vi "期末9-2.vi"() -> ()   [LabVIEW 2014]
uses:
  <vilib>/vision/NI_Vision_Development_Module.lvlib
panel:
  out "Image Out 2":T1(plugin-control)
  out "ROI":T2
  in  "紀錄中點座標和":bool
  out "填入飽和磁場分量尖點座標和 2":dbl
  out "填入飽和磁場分量尖點座標和平均 2":dbl
  in  "3. Number of Erosion":i32=10
  out "Image Out":T1(plugin-control)
  in  "紀錄電流":dbl[](array[numeric])
  in  "Tab Control 2":enum32{"座標", "座標和", "作圖"}(tab)
  out "瞬間尖點座標":dbl[][](array[numeric])
  out "尖點座標和":dbl[](array[numeric])
  out "相減結果":dbl[](array[numeric])
  out "分量-電流":cluster{"紀錄電流":dbl[], dbl[]}(graph)
  in  "紀錄":bool
  in  "結束實驗":bool
  in  "1. 範圍選擇":T3={"色相（H）"={0, 255}, "飽和度（S）"={0, 255}, "亮度（L）"={0, 255}} {"亮度（L）" scale=0.0..255.0; "飽和度（S）" scale=0.0..255.0; "色相（H）" scale=0.0..255.0}
  out "Number of Particles":i32
  out "output cluster":cluster{"X":dbl, "Y":dbl}
  in  "Tab Control":T4(tab)
  out "1. 顏色選取":T1(plugin-control)
  out "2. 填補空隙":T1(plugin-control)
  out "3. 移除雜點":T1(plugin-control)
  out "4. 形狀修正":T1(plugin-control)
  out "5. 選取結果":T1(plugin-control)
  out "Particle Measurements":dbl[][](array[numeric])
  out "Error Out":errorcluster
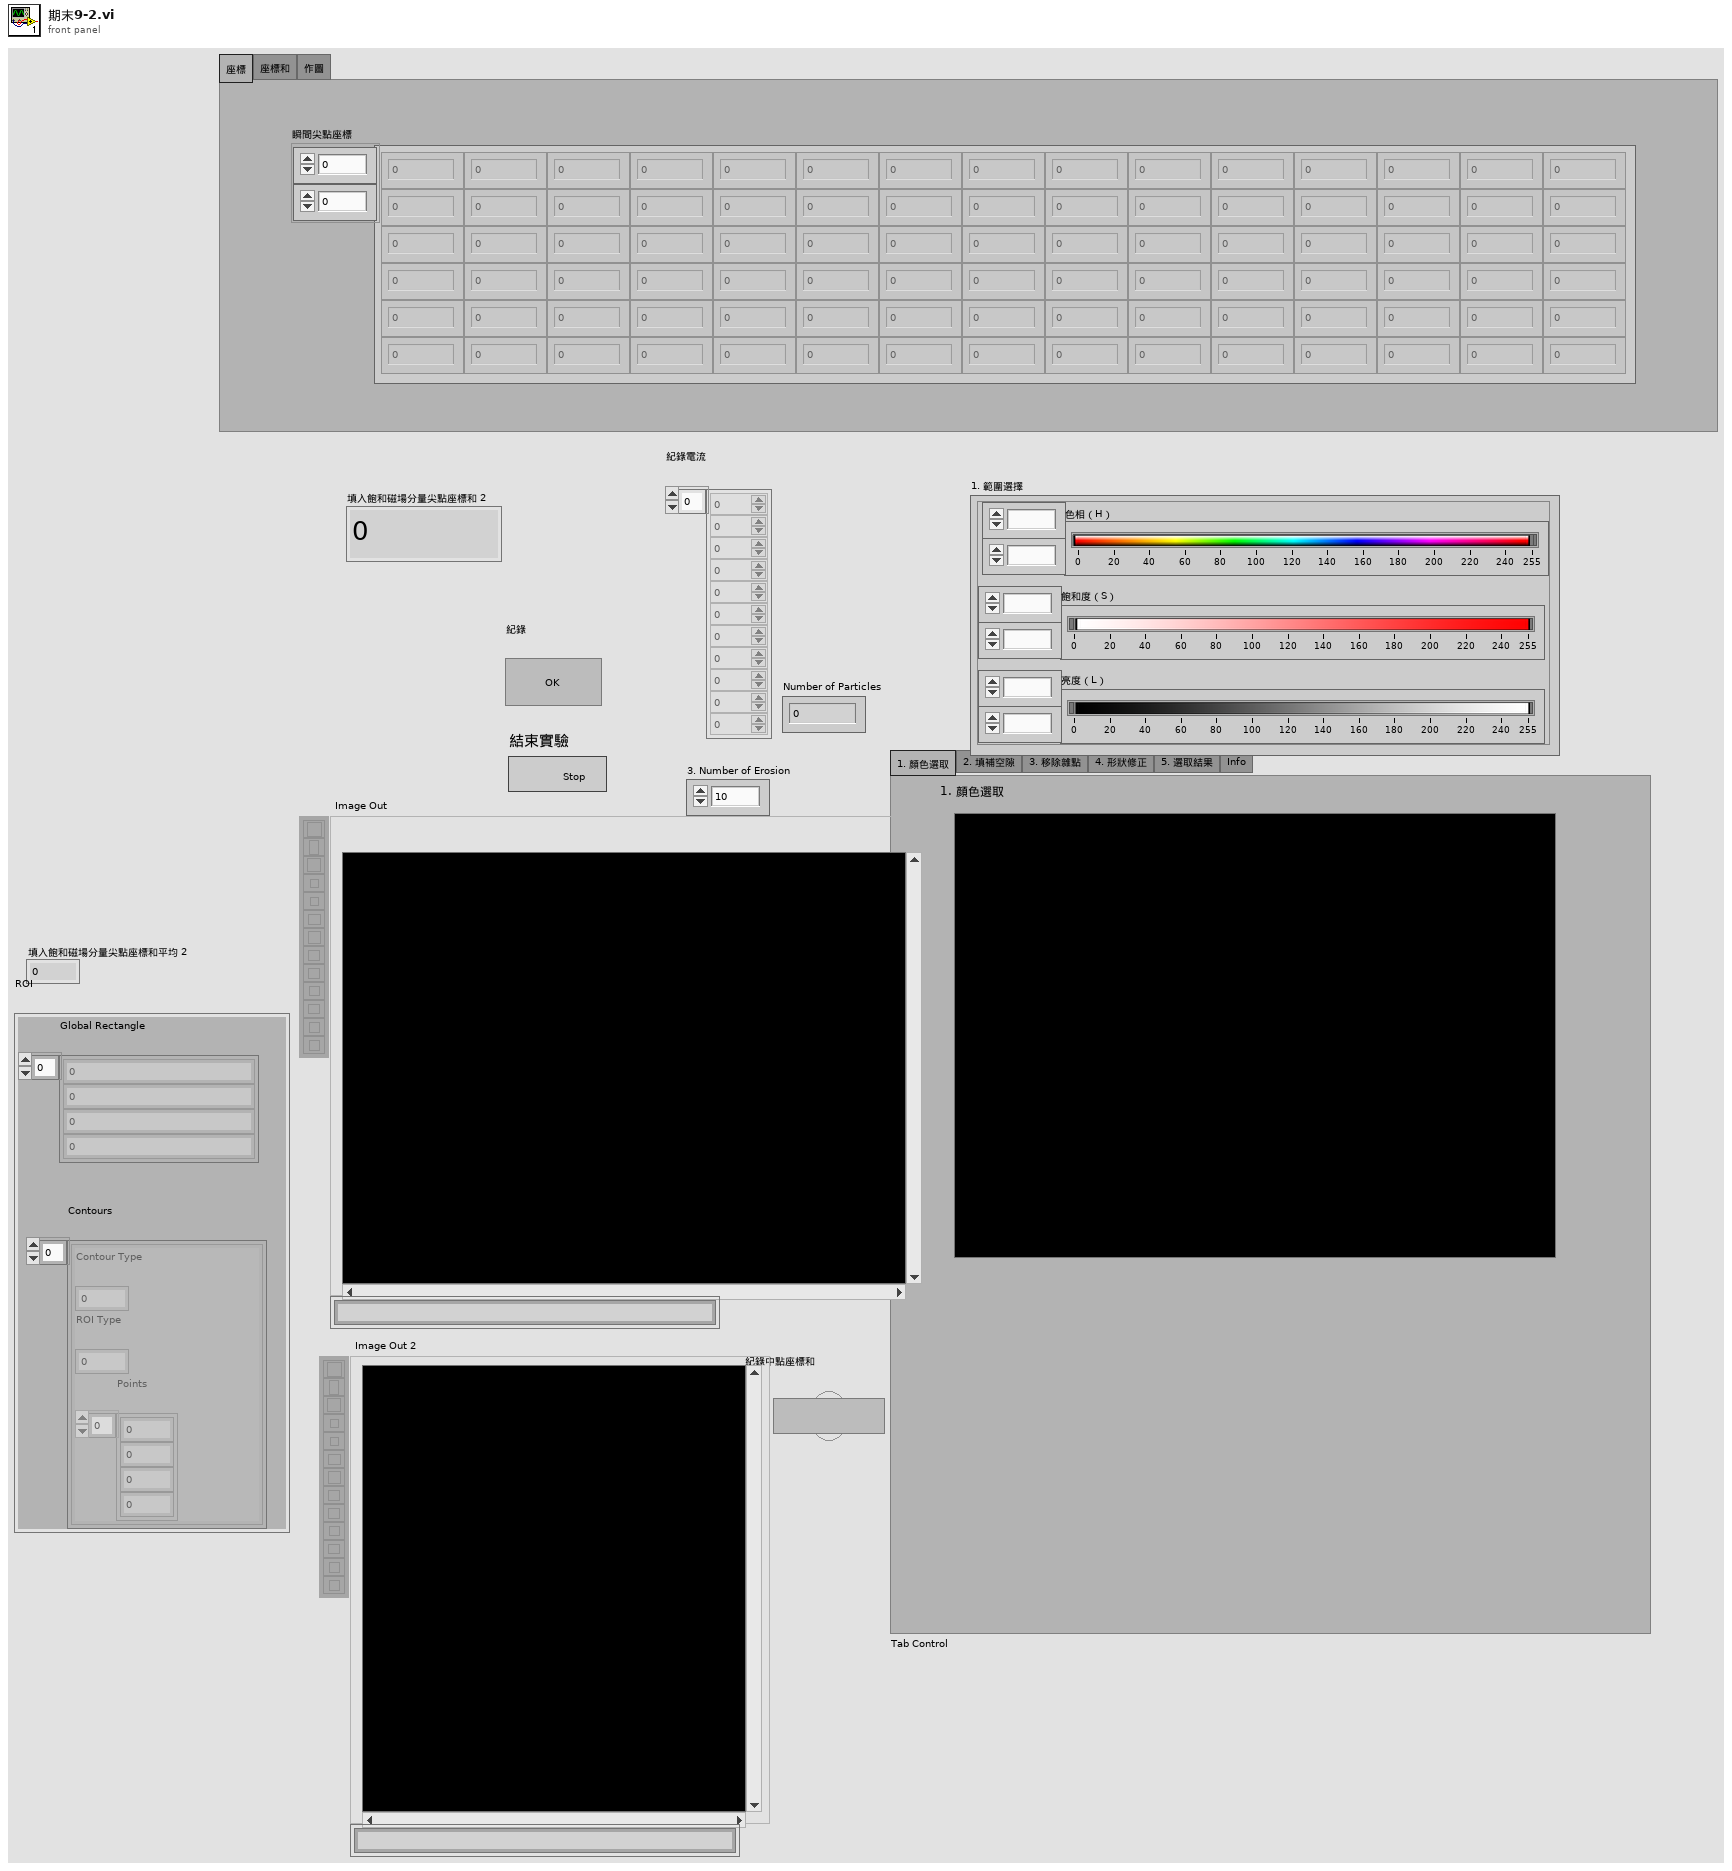
[diagram p1: front panel]
types:
  T1 = typedef "IMAQ Image.ctl" = refnum<image>
  T2 = cluster{"Global Rectangle":i32[], "Contours":cluster{"Contour Type":u32, "ROI Type":u32, "Points":i32[]}[]}
  T3 = cluster{"色相（H）":cluster{u8, u8}, "飽和度（S）":cluster{u8, u8}, "亮度（L）":cluster{u8, u8}}
  T4 = enum32{"1. 顏色選取", "2. 填補空隙", "3. 移除雜點", "4. 形狀修正", "5. 選取結果", "Info"}
  T5 = typedef "Image Type" = u32
  T6 = cluster{"Numeric":dbl, "Numeric":dbl, "Numeric":dbl, "Numeric":dbl}
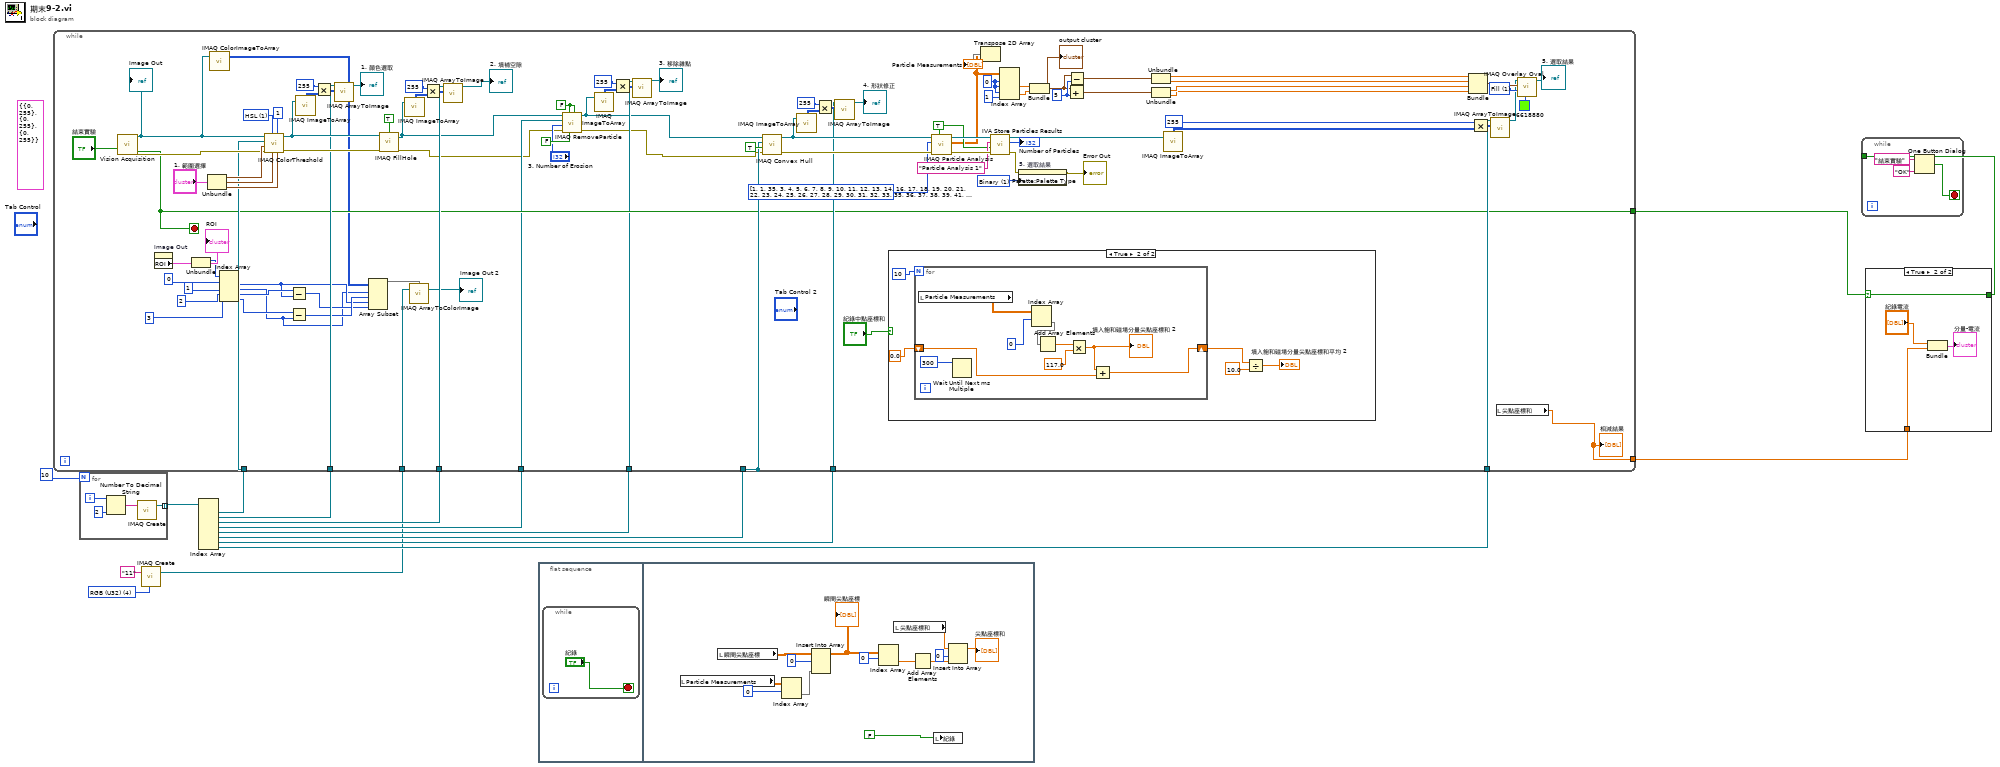
[diagram p0: block diagram]
diagram:
  w2 = T5 4 items=["Grayscale (U8)", "Grayscale (I16)", "Grayscale (SGL)", "Complex (CSG)", "RGB (U32)", "HSL (U32)", "RGB (U64)", "Grayscale (U16)"] ("Image Type")
  (unwired) T3 {"色相（H）"={0, 255}, "飽和度（S）"={0, 255}, "亮度（L）"={0, 255}} ("範圍選擇")
  n1 = for {
    N: 10 -> [_]
    tunnel: [w17] -> w16 mode=indexing
    i -> [w19]
    n2 = Number To Decimal String(number=w19, width (-)=2) -> (decimal integer string=w18:string)
    n3 = call "IMAQ Create"("Image Name"=w18) -> ("New Image"=w17:T1)  [unwired: 4 in, 1 out]
  }
  n4 = call "IMAQ Create"("Image Name"="11", "Image Type"=w2) -> ("New Image"=w3:T1)  [unwired: 3 in, 1 out]
  n5 = Index Array(array=w16) -> (element #1=w15:T1, element #2=w14:T1, element #3=w13:T1, element #4=w5:T1, element #5=w4:T1, element #6=w11:T1, element #7=w10:T1, element #8=w9:T1)  [unwired: 8 in]
  n6 = while {
    tunnel: w13 -> [w87]
    tunnel: w11 -> [w98]
    tunnel: [w98] -> _
    tunnel: w14 -> [w92]
    tunnel: w15 -> [w86]
    tunnel: w10 -> [w80]
    tunnel: w9 -> [w57]
    tunnel: [w53] -> w8
    tunnel: [w39] -> w6
    tunnel: w5 -> [w46]
    tunnel: w4 -> [w45]
    tunnel: w3 -> [w29]
    stop <- w53 stop-if-true
    w50 = FALSE ("Connectivity 4/8 (8)")
    w62 = u32 1 items=["Frame", "Fill"] ("Drawing Mode (Frame)")
    w71 = 5
    w76 = 0
    w100 = u32 1 items=["Grayscale", "Binary", "Gradient", "Rainbow", "Temperature", "User Defined"] ("Palette")
    w105 = i32[] [1, 1, 35, 3, 4, 5, 6, 7, 8, 9, 10, 11, 12, 13, 14, 16, 17, 18, 19, 20, 21, 22, 23, 24, 25, 26, 27, 28, 29, 30, 31, 32, 33, 35, 36, 37, 38, 39, 41, 42, 43, 45, 46, 48, 49, 50, 51, 53, 54, 55, 56, 58, 59, 60, 61, 62, 63, 64, 65, 66, 68, 69, 70, 71, 72, 73, 74, 75, 76, 77, 78, 79, 80, 81, 82, 83, 84, 85, 86, 87, 88] items=["Center of Mass X", "Center of Mass Y", "First Pixel X", "First Pixel Y", "Bounding Rect Left", "Bounding Rect Top", "Bounding Rect Right", "Bounding Rect Bottom", "Max Feret Diameter Start X", "Max Feret Diameter Start Y", "Max Feret Diameter End X", "Max Feret Diameter End Y", "Max Horiz. Segment Length Left", "Max Horiz. Segment Length Right", "Max Horiz. Segment Length Row", "-", "Bounding Rect Width", "Bounding Rect Height", "Bounding Rect Diagonal", "Perimeter", "Convex Hull Perimeter", "Holes' Perimeter", "Max Feret Diameter", "Equivalent Ellipse Major Axis", "Equivalent Ellipse Minor Axis", "Equivalent Ellipse Minor Axis (Feret)", "Equivalent Rect Long Side", "Equivalent Rect Short Side", "Equivalent Rect Diagonal", "Equivalent Rect Short Side (Feret)", "Average Horiz. Segment Length", "Average Vert. Segment Length", "Hydraulic Radius", "Waddel Disk Diameter", "-", "Area", "Holes' Area", "Particle & Holes' Area", "Convex Hull Area", "Image Area", "-", "Number of Holes", "Number of Horiz. Segments", "Number of Vert. Segments", "-", "Orientation", "Max Feret Diameter Orientation", "-", "% Area/Image Area", "% Area/(Particle & Holes' Area)", "Ratio of Equivalent Ellipse Axes", "Ratio of Equivalent Rect Sides", "-", "Elongation Factor", "Compactness Factor", "Heywood Circularity Factor", "Type Factor", "-", "Sum X", "Sum Y", "Sum XX", "Sum XY", "Sum YY", "Sum XXX", "Sum XXY", "Sum XYY", "Sum YYY", "-", "Moment of Inertia XX", "Moment of Inertia XY", "Moment of Inertia YY", "Moment of Inertia XXX", "Moment of Inertia XXY", "Moment of Inertia XYY", "Moment of Inertia YYY", "Norm. Moment of Inertia XX", "Norm. Moment of Inertia XY", "Norm. Moment of Inertia YY", "Norm. Moment of Inertia XXX", "Norm. Moment of Inertia XXY", "Norm. Moment of Inertia XYY", "Norm. Moment of Inertia YYY", "Hu Moment 1", "Hu Moment 2", "Hu Moment 3", "Hu Moment 4", "Hu Moment 5", "Hu Moment 6", "Hu Moment 7"] ("Pixel Measurements")
    w107 = TRUE ("Connectivity 4/8 (8)")
    w116 = u16 1 items=["RGB", "HSL", "HSV", "HSI"] ("Color Mode")
    n7 = call "Vision Acquisition"("Stop (F)"="結束實驗") -> ("Image Out"=w37:T1, "Stopped"=w53:bool, "error out"=w111:errorcluster)  [unwired: 24 in]
    "Image Out" <- w37
    n8 = property on="Image Out" class="ImageControl"() -> ("ROI"=w35:T2)  [unwired: 2 in, 2 out]
    "ROI" <- w35
    n9 = Unbundle(w35) -> ("Global Rectangle"=w34:i32[])  [unwired: 1 out]
    n10 = Unbundle("1. 範圍選擇") -> ("色相（H）"=w115:cluster{u8, u8}, "飽和度（S）"=w114:cluster{u8, u8}, "亮度（L）"=w113:cluster{u8, u8})
    n11 = call "IMAQ ColorImageToArray"("Image"=w37) -> ("Image Pixels (U32)"=w36:u32[][])  [unwired: 3 in, 2 out]
    n12 = Index Array(array=w34, index #1=0 ("index"), index #2=1 ("index"), index #3=2 ("index"), index #4=3 ("index")) -> (element #1=w23:i32, element #2=w21:i32, element #3=w26:i32, element #4=w22:i32)
    n13 = call "IMAQ ColorThreshold"("Blue or Luma or Val or Inten Range"=w113, "Replace Value"=1, "Green or Sat Range"=w114, "Color Mode"=w116, "error in (no error)"=w111, "Red or Hue Range"=w115, "Image Dst"=w86, "Image Src"=w37) -> ("error out"=w102:errorcluster, "Image Dst Out"=w97:T1)  [unwired: 2 out]
    n14 = Subtract(x=w26, y=w23) -> (x-y=w24:i32)
    n15 = Subtract(x=w22, y=w21) -> (x-y=w25:i32)
    n16 = call "IMAQ ImageToArray"("Image"=w97) -> ("Image Pixels (U8)"=w95:u8[][])  [unwired: 3 in, 4 out]
    n17 = Multiply(x=255, y=w95) -> (x*y=w94:i32[][])
    n18 = call "IMAQ ArrayToImage"("Image Pixels (U8)"=w94, "Image"=w92) -> ("Image Out"=→"1. 顏色選取":T1)  [unwired: 8 in, 1 out]
    n19 = Array Subset(array=w36, index (row)=w21, length (row)=w25, index (col)=w23, length (col)=w24) -> (w27:u32[][])
    n20 = call "IMAQ FillHole"("error in (no error)"=w102, "Image Src"=w97, "Connectivity 4/8 (8)"=TRUE) -> ("error out"=w44:errorcluster, "Image Dst Out"=w42:T1)  [unwired: 1 in, 2 out]
    n21 = call "IMAQ ImageToArray"("Image"=w42) -> ("Image Pixels (U8)"=w90:u8[][])  [unwired: 3 in, 4 out]
    n22 = call "IMAQ ArrayToColorImage"("Image Pixels (U32)"=w27, "Image"=w29) -> ("Image Out"=→"Image Out 2":T1)  [unwired: 3 in, 1 out]
    n23 = Multiply(x=255, y=w90) -> (x*y=w91:i32[][])
    n24 = call "IMAQ ArrayToImage"("Image Pixels (U8)"=w91, "Image"=w87) -> ("Image Out"=→"2. 填補空隙":T1)  [unwired: 8 in, 1 out]
    n25 = call "IMAQ RemoveParticle"("Connectivity 4/8 (8)"=w50, "Low Pass/High Pass (Low)"=FALSE, "Square/Hexa (Square)"=w50, "error in (no error)"=w44, "Number of Erosion"="3. Number of Erosion", "Image Dst"=w46, "Image Src"=w42) -> ("error out"=w43:errorcluster, "Image Dst Out"=w41:T1)  [unwired: 3 out]
    n26 = call "IMAQ ImageToArray"("Image"=w41) -> ("Image Pixels (U8)"=w40:u8[][])  [unwired: 3 in, 4 out]
    n27 = Multiply(x=255, y=w40) -> (x*y=w48:i32[][])
    n28 = call "IMAQ ArrayToImage"("Image Pixels (U8)"=w48, "Image"=w45) -> ("Image Out"=→"3. 移除雜點":T1)  [unwired: 8 in, 1 out]
    n29 = call "IMAQ Convex Hull"("error in (no error)"=w43, "Connectivity 4/8 (8)"=TRUE, "Image Dst"=w98, "Image Src"=w41) -> ("error out"=w106:errorcluster, "Image Dst Out"=w81:T1)  [unwired: 6 out]
    n30 = call "IMAQ ImageToArray"("Image"=w81) -> ("Image Pixels (U8)"=w84:u8[][])  [unwired: 3 in, 4 out]
    n31 = Multiply(x=255, y=w84) -> (x*y=w85:i32[][])
    n32 = call "IMAQ ArrayToImage"("Image Pixels (U8)"=w85, "Image"=w80) -> ("Image Out"=→"4. 形狀修正":T1)  [unwired: 8 in, 1 out]
    n33 = case shown="True" "紀錄中點座標和" {
      frame False {
      }
      frame True {
        n34 = for {
          N: 10 -> [_]
          shift-right: [w123] -> w120
          shift-left: 0.0 -> [w125]
          n35 = local read "Particle Measurements"() -> (w130:dbl[][])
          n36 = Wait Until Next ms Multiple(millisecond multiple=u32 300 ("millisecond timer value")) -> ()  [unwired: 1 out]
          n37 = Index Array(array=w130, index (row)=0) -> (element=w129:dbl[])  [unwired: 1 in]
          n38 = Add Array Elements(numeric array=w129) -> (sum=w128:dbl)
          n39 = Multiply(x=w128, y=117.0) -> (x*y=w124:dbl)
          "填入飽和磁場分量尖點座標和 2" <- w124
          n40 = Add(x=w124, y=w125) -> (x+y=w123:dbl)
        }
        n41 = Divide(x=w120, y=10.0) -> (x/y=→"填入飽和磁場分量尖點座標和平均 2":dbl)
      }
    }
    n42 = call "IMAQ Particle Analysis"("Connectivity 4/8 (8)"=w107, "error in (no error)"=w106, "Pixel Measurements"=w105, "Image"=w81) -> ("error out"=w110:errorcluster, "Particle Measurements (Pixels)"=w77:dbl[][], "Image Out (duplicate)"=w108:T1)  [unwired: 1 in, 4 out]
    n43 = Transpose 2D Array(2D array=w77) -> (transposed array=→"Particle Measurements":dbl[][])
    n44 = call <vilib>:"IVA Store Particles Results.vi"("error in (no error)"=w110, "Connectivity 4/8 (8)"=w107, "Step Name"="Particle Analysis 1", "Image in"=w108) -> ("error out"=w101:errorcluster, "Number of Particles"=→"Number of Particles":i32, "Image dup"=w61:T1)  [unwired: 5 out]
    n45 = Index Array(array=w77, index (row) #1=w76, index (col) #1=w76, index (row) #2=w76, index (col) #2=1) -> (element #1=w74:dbl, element #2=w73:dbl)
    n46 = property on="5. 選取結果" class="ImageControl"(error in=w101, "Palette:Palette Type"=w100) -> (error out=→"Error Out":errorcluster)  [unwired: 1 in, 1 out]
    n47 = Bundle("Numeric"=w74, "Numeric"=w73) -> (w70:cluster{"Numeric":dbl, "Numeric":dbl})  [unwired: 1 in]
    "output cluster" <- w70
    n48 = Add(x=w70, y=w71) -> (x+y=w68:cluster{"Numeric":dbl, "Numeric":dbl})
    n49 = Subtract(x=w70, y=w71) -> (x-y=w69:cluster{"Numeric":dbl, "Numeric":dbl})
    n50 = Unbundle(w69) -> ("Numeric"=w67:dbl, "Numeric"=w66:dbl)
    n51 = Unbundle(w68) -> ("Numeric"=w65:dbl, "Numeric"=w64:dbl)
    n52 = call "IMAQ ImageToArray"("Image"=w61) -> ("Image Pixels (U8)"=w58:u8[][])  [unwired: 3 in, 4 out]
    n53 = Bundle("Numeric"=w67, "Numeric"=w66, "Numeric"=w65, "Numeric"=w64) -> (w63:T6)  [unwired: 1 in]
    n54 = Multiply(x=255, y=w58) -> (x*y=w59:i32[][])
    n55 = call "IMAQ ArrayToImage"("Image Pixels (U8)"=w59, "Image"=w57) -> ("Image Out"=w56:T1)  [unwired: 8 in, 1 out]
    n56 = local read "尖點座標和"() -> (w39:dbl[])
    "相減結果" <- w39
    n57 = call "IMAQ Overlay Oval"("Color"=u32 6618880, "Drawing Mode (Frame)"=w62, "Bounding Rectangle"=w63, "Image"=w56) -> ("Image Out"=→"5. 選取結果":T1)  [unwired: 6 in, 1 out]
  }
  n58 = flat-sequence {
    frame #0 {
      n59 = while {
        stop <- "紀錄" stop-if-true
      }
    }
    frame #1 {
      n60 = local read "Particle Measurements"() -> (w134:dbl[][])
      n61 = local read "瞬間尖點座標"() -> (w140:dbl[][])
      n62 = Index Array(array=w134, index (row)=0) -> (element=w139:dbl[])  [unwired: 1 in]
      n63 = Insert Into Array(array=w140, index (row)=0 ("index"), new element=w139) -> (w142:dbl[][])  [unwired: 1 in]
      "瞬間尖點座標" <- w142
      n64 = Index Array(array=w142, index (row)=0) -> (element=w144:dbl[])  [unwired: 1 in]
      n65 = local read "尖點座標和"() -> (w135:dbl[])
      n66 = Add Array Elements(numeric array=w144) -> (sum=w137:dbl)
      n67 = local write "紀錄"(FALSE) -> ()
      n68 = Insert Into Array(array=w135, index=0 ("index (row)"), new element=w137) -> (→"尖點座標和":dbl[])
    }
  }
  n69 = case shown="True" w8 {
    selector: w8 -> [w146 w150]
    tunnel: [w146 w150] -> w7
    tunnel: w6 -> [_ w149]
    frame False {
    }
    frame True {
      n70 = Bundle("紀錄電流"="紀錄電流", "尖點座標和"=w149) -> (→"分量-電流":cluster{"紀錄電流":dbl[], "尖點座標和":dbl[]})  [unwired: 1 in]
    }
  }
  n71 = while {
    tunnel: w7 -> [_]
    stop <- w153 stop-if-true
    n72 = One Button Dialog(message="結束實驗", button name ("OK")="OK") -> (true=w153:bool)
  }
